vi "Get Log Specification Type.vi"(8 "error in (no error)":errorcluster, 11 "Log File Specification in":refnum<class "Log File Specification.lvclass">) -> (0 "error out":errorcluster, 2 "Log Specification Type":T1, 3 "Log File Specification out":refnum<class "Log File Specification.lvclass">)   [LabVIEW 2015, in "Waveform Data Logger Shared.lvlib" / "Log File Specification.lvclass"]
uses:
  Log File Specification.lvclass
  Log Specification Type.ctl
  Log File Specification.lvclass/Log File Specification.ctl
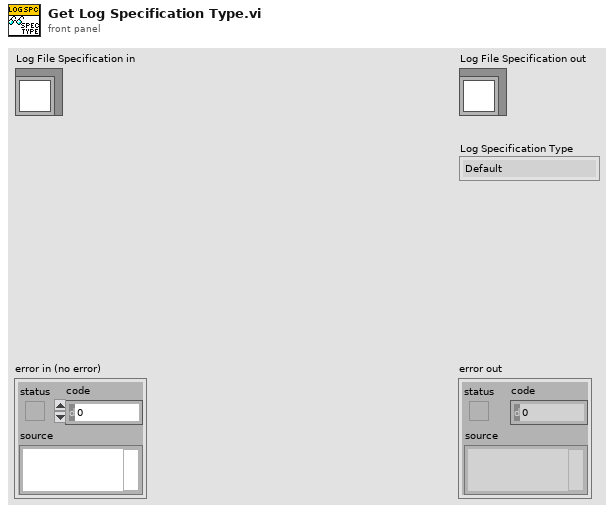
[diagram p1: front panel]
types:
  T1 = typedef "Waveform Data Logger Shared.lvlib/Log File Specification.lvclass/Log Specification Type.ctl" = enum16{"Default", "TDMS", "Text", "Waveform TDMS"}
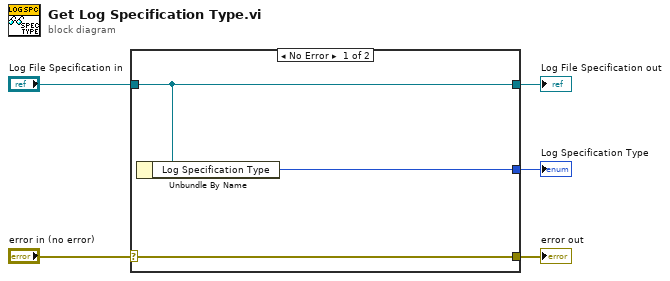
[diagram p0: block diagram]
diagram:
  n1 = case shown="No Error" "error in (no error)" {
    selector: "error in (no error)" -> [w8 w9]
    tunnel: [w8 w9] -> w4
    tunnel: [w7 w10] -> w2
    tunnel: "Log File Specification in" -> [w7 w10]
    tunnel: [w6 _] -> w1
    frame No Error {
      n2 = Unbundle By Name(w7) -> ("Log Specification Type"=w6:T1)
    }
    frame Error {
    }
  }
  "error out" <- w4
  "Log File Specification out" <- w2
  "Log Specification Type" <- w1
